vi "Random Command Generator.vi"(7 "Command Array":string[](array[string])=["Velocity Move", "ABS Pos Move", "REL Pos Move", "Stop"], 8 "error in (no error)":errorcluster, 9 "Motion Parameters (Min)":T2={"position"=0.0, "velocity"=0.0, "acceleration"=80000.0, "deceleration"=80000.0, "accel. jerk"=80000.0, "decel. jerk"=80000.0}, 10 "Motion Parameters (Max)":T2={"position"=10000.0, "velocity"=10000.0, "acceleration"=100000.0, "deceleration"=100000.0, "accel. jerk"=100000.0, "decel. jerk"=100000.0}, 11 "Axis Resources":refnum<k21>[](array[refnum])=["Axis 1", "Axis 2", "Axis 3", "Axis 4", "Axis 5", "Axis 6", "Axis 7", "Axis 8"]) -> (0 "error out":errorcluster, 1 "Motor_Message":T1={"Axis"="Axis 1", "Motion Parameters"={"position"=1000.0, "velocity"=1000.0, "acceleration"=10000.0, "deceleration"=10000.0, "accel. jerk"=10000.0, "decel. jerk"=10000.0}}, 2 "Command Out":string)   [LabVIEW 2013]
doc: "Generates random commands given max and min limits."
uses:
  EMC API/EMC_Typedef_Motor_Parameters.ctl
  Typedef/Typedef_Motor_Message.ctl
panel:
  out "Random Motion":T2={"position"=750.2770424000067, "velocity"=961.5177141839189, "acceleration"=8853.399008279855, "deceleration"=9726.007423274288, "accel. jerk"=9637.260136271336, "decel. jerk"=8268.625053543105}
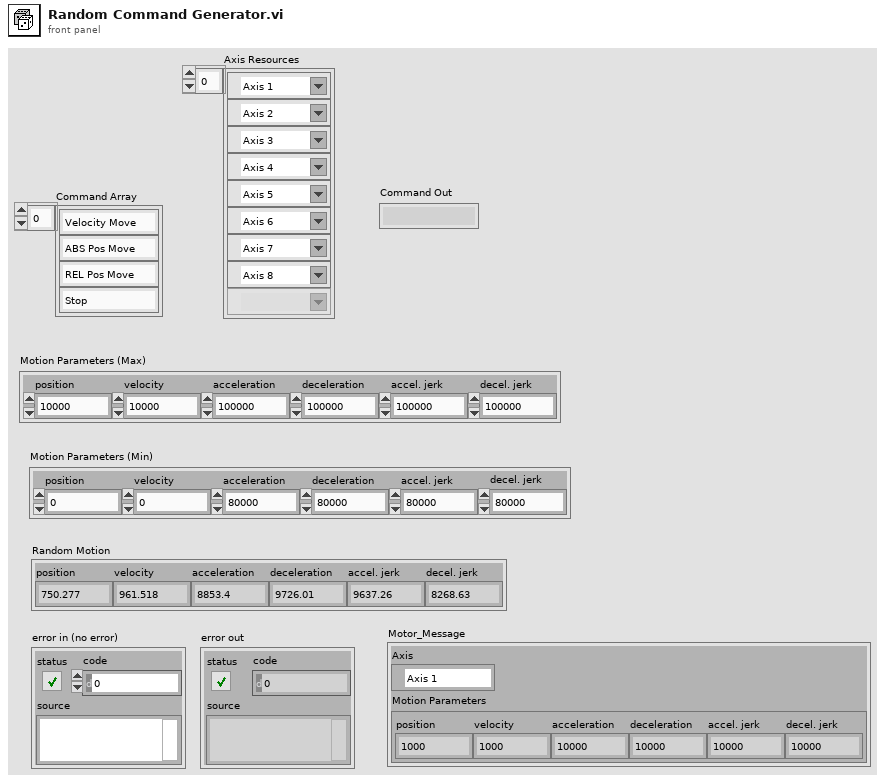
[diagram p1: front panel]
types:
  T1 = typedef "Typedef_Motor_Message.ctl" = cluster{"Axis":refnum<k21>, "Motion Parameters":T2}
  T2 = typedef "EMC_Typedef_Motor_Parameters.ctl" = cluster{"position":dbl, "velocity":dbl, "acceleration":dbl, "deceleration":dbl, "accel. jerk":dbl, "decel. jerk":dbl}
  T3 = cluster{"[0]":dbl, "[1]":dbl, "[2]":dbl, "[3]":dbl, "[4]":dbl, "[5]":dbl}
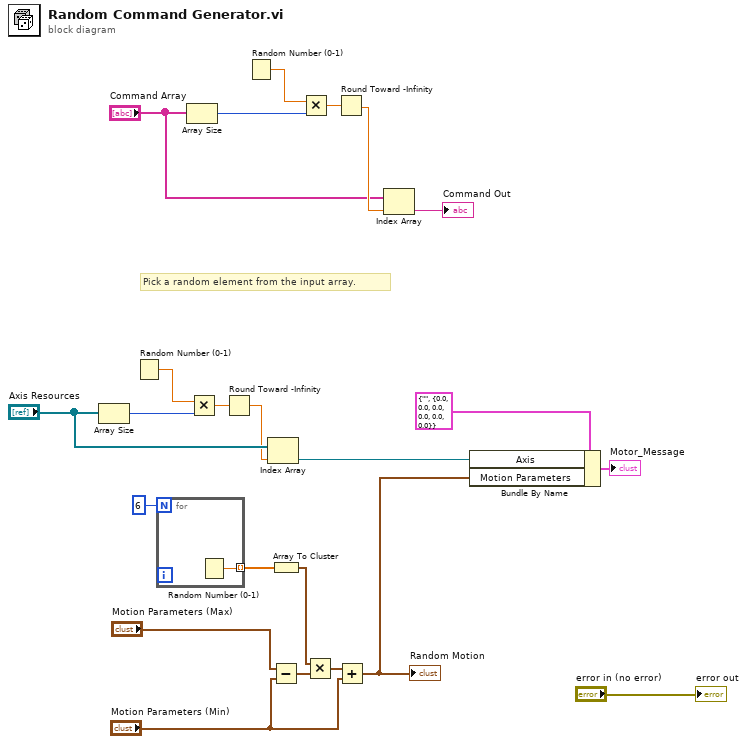
[diagram p0: block diagram]
diagram:
  # "Pick a random element from the input array."
  n1 = Array Size(array="Axis Resources") -> (size(s)=w5:i32)
  n2 = Random Number (0-1)() -> (number: 0 to 1=w6:dbl)
  n3 = for {
    N: 6 -> [_]
    tunnel: [w24] -> w21 mode=indexing
    n4 = Random Number (0-1)() -> (number: 0 to 1=w24:dbl)
  }
  n5 = Array Size(array="Command Array") -> (size(s)=w15:i32)
  n6 = Multiply(x=w6, y=w5) -> (x*y=w4:dbl)
  n7 = Round Toward -Infinity(1:w4) -> (0:w2:dbl)
  n8 = Random Number (0-1)() -> (number: 0 to 1=w16:dbl)
  n9 = Index Array(array="Axis Resources", index=w2) -> (element=w1:refnum<k21>)
  n10 = Array To Cluster(array=w21) -> (cluster=w20:T3)
  n11 = Subtract(x="Motion Parameters (Max)", y="Motion Parameters (Min)") -> (x-y=w19:T2)
  n12 = Multiply(x=w16, y=w15) -> (x*y=w14:dbl)
  n13 = Multiply(x=w20, y=w19) -> (x*y=w18:T2)
  n14 = Round Toward -Infinity(1:w14) -> (0:w13:dbl)
  n15 = Add(x=w18, y="Motion Parameters (Min)") -> (x+y=w8:T2)
  "Random Motion" <- w8
  n16 = Index Array(array="Command Array", index=w13) -> (element=→"Command Out":string)
  n17 = Bundle By Name(cluster=T1 {"Axis"="", "Motion Parameters"={"position"=0.0, "velocity"=0.0, "acceleration"=0.0, "deceleration"=0.0, "accel. jerk"=0.0, "decel. jerk"=0.0}} ("Motor_Message"), "Axis"=w1, "Motion Parameters"=w8) -> (→"Motor_Message":T1)
  "error out" <- "error in (no error)"
